vi "case stru ( factorial).vi"() -> ()   [LabVIEW 2014]
panel:
  out "Numeric":dbl format="%#_13g"
  in  "input":dbl format="%#_13g"
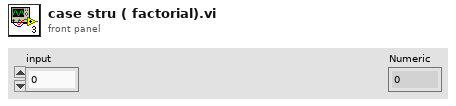
[diagram p1: front panel]
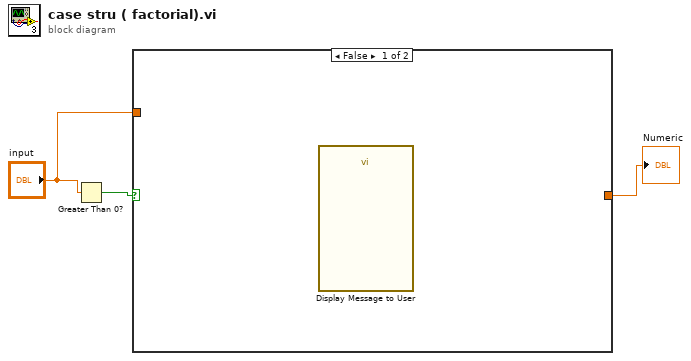
[diagram p0: block diagram]
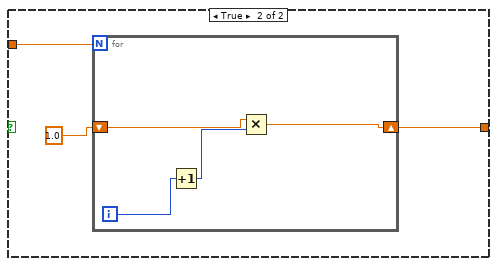
[diagram p2: hidden frame]
diagram:
  n1 = Greater Than 0?(x="input") -> (x > 0?=w3:bool)
  n2 = case shown="False" w3 {
    tunnel: "input" -> [_ w5]
    tunnel: [_ w4] -> w1
    frame False {
      n3 = call "Display Message to User"() -> ()  [unwired: 10 in, 2 out]
    }
    frame True {
      n4 = for {
        N: w5 -> [_]
        shift-right: [w7] -> w4
        shift-left: 1.0 -> [w10]
        i -> [w8]
        n5 = Increment(x=w8) -> (x+1=w9:i32)
        n6 = Multiply(x=w10, y=w9) -> (x*y=w7:dbl)
      }
    }
  }
  "Numeric" <- w1
